vi "SRV_Read 12 Bytes of Data.vi"(8 "error in (no error)":errorcluster, 11 "SRV In":refnum<k5>) -> (0 "error out":errorcluster, 1 "Data out":string, 3 "SRV Out":refnum<k5>, 5 "Read more data":bool)   [LabVIEW 2009]
doc: "Samples the data available on the SRV's serial line. Indicates the type of data (text vs image).\n\nCreated for Benilde St. Margaret's School - Tim Jump\nBy Doug Schmertman - Logic PD\nCopyright 2012"
uses:
  TCP_Communication/SRV_TCP Settings.ctl
  TCP_Communication/SRV_Package Methods.ctl
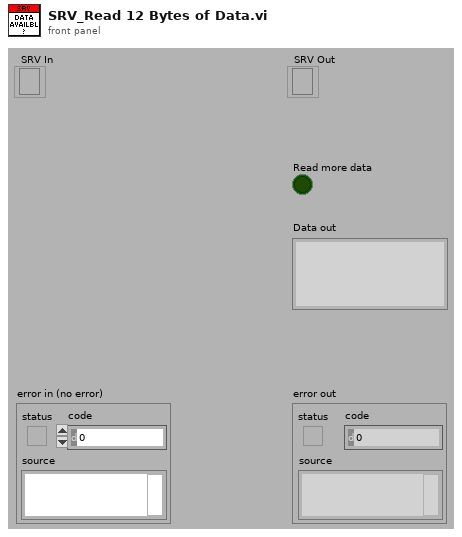
[diagram p1: front panel]
types:
  T1 = typedef "SRV_TCP Settings.ctl" = cluster{"Method":T2, "bytes to read":i32, "timeout ms (1000)":i32}
  T2 = typedef "SRV_Package Methods.ctl" = enum16{"General", "Standard", "CRLF", "Image", "HTML"}
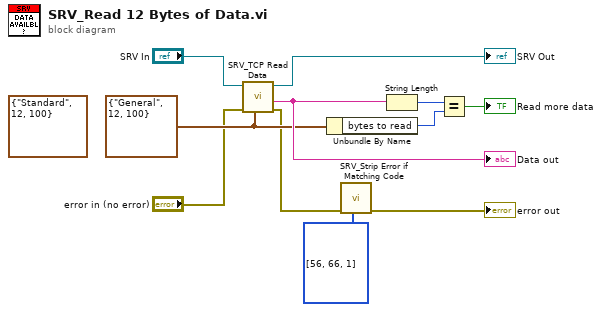
[diagram p0: block diagram]
diagram:
  (unwired) T1 {"Method"=enum."Standard", "bytes to read"=12, "timeout ms (1000)"=100} ("TCP Settings")
  w3 = T1 {"Method"=enum."General", "bytes to read"=12, "timeout ms (1000)"=100} ("TCP Settings")
  n1 = call "SRV_TCP Read Data.vi"("TCP Settings"=w3, "error in"="error in (no error)", "connection ID in"="SRV In") -> ("error out"=w1:errorcluster, "data out"=w4:string, "connection ID"=→"SRV Out":refnum<k5>)  [unwired: 2 in, 1 out]
  "Data out" <- w4
  n2 = Unbundle By Name(w3) -> ("bytes to read"=w8:i32)
  n3 = call "SRV_Strip Error if Matching Code.vi"("error in (no error)"=w1, "Strip Codes"=i32[] [56, 66, 1]) -> ("error out"=→"error out":errorcluster)  [unwired: 8 in]
  n4 = String Length(string=w4) -> (length=w11:i32)
  n5 = Equal?(x=w11, y=w8) -> (x = y?=→"Read more data":bool)
